vi "subFixUpLooseFiles.vi"(8 "error in (no error)":errorcluster, 9 "Loose files":path[](array[path])=[path "E:/Repos/LVDependencyInspector/obj/DependencyInspector.vi"], 10 "Dependency order":T1[](array[typedef])=[{"Library ref"=refnum, "Target path"=path "E:/Repos/LVDependencyInspector/obj/Addons/LabVIEWObjectInterfaces.lvlibp", "Source name"="LabVIEWObjectInterfaces.lvlib", "Build spec name"="LabVIEWObjectInterfaces"}, {"Library ref"=refnum, "Target path"=path "E:/Repos/LVDependencyInspector/obj/Addons/ErrorManager.lvlibp", "Source name"="ErrorManager.lvlib", "Build spec name"="ErrorManager"}, {"Library ref"=refnum, "Target path"=path "E:/Repos/LVDependencyInspector/obj/Addons/ExtensionInterfaces.lvlibp", "Source name"="ExtensionInterfaces.lvlib", "Build spec name"="ExtensionInterfaces"}, {"Library ref"=refnum, "Target path"=path "E:/Repos/LVDependencyInspector/obj/Addons/LabVIEWItem.lvlibp", "Source name"="LabVIEWItem.lvlib", "Build spec name"="LabVIEWItem"}, {"Library ref"=refnum, "Target path"=path "E:/Repos/LVDependencyInspector/obj/Addons/DefaultExtensions.lvlibp", "Source name"="DefaultExtensions.lvlib", "Build spec name"="DefaultExtensions"}, {"Library ref"=refnum, "Target path"=path "E:/Repos/LVDependencyInspector/obj/Addons/LabVIEWContainers.lvlibp", "Source name"="LabVIEWContainers.lvlib", "Build spec name"="LabVIEWContainers"}, {"Library ref"=refnum, "Target path"=path "E:/Repos/LVDependencyInspector/obj/Addons/LabVIEWFiles.lvlibp", "Source name"="LabVIEWFiles.lvlib", "Build spec name"="LabVIEWFiles"}, {"Library ref"=refnum, "Target path"=path "E:/Repos/LVDependencyInspector/obj/Addons/LabVIEWObjectFactory.lvlibp", "Source name"="LabVIEWObjectFactory.lvlib", "Build spec name"="LabVIEWObjectFactory"}, {"Library ref"=refnum, "Target path"=path "E:/Repos/LVDependencyInspector/obj/Addons/DependencyInspection.lvlibp", "Source name"="DependencyInspection.lvlib", "Build spec name"="DependencyInspection"}, {"Library ref"=refnum, "Target path"=path "E:/Repos/LVDependencyInspector/obj/Addons/DependencyInspector.lvlibp", "Source name"="DependencyInspector.lvlib", "Build spec name"="DependencyInspector"}, {"Library ref"=refnum, "Target path"=path "", "Source name"="Application", "Build spec name"="Application"}], 11 "Local Host App Instance":refnum<vi>) -> (0 "error out":errorcluster)   [LabVIEW 2020, in "SolutionBuilder.lvlib" / "SolutionBuilder.lvclass"]
uses:
  SolutionBuilder.lvclass
  Private/FileInfo.ctl
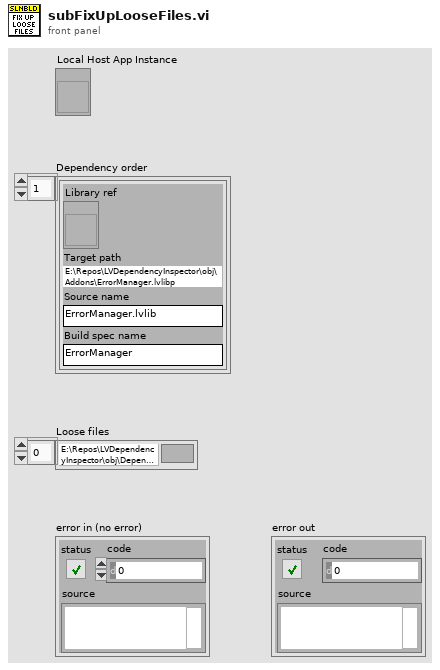
[diagram p1: front panel]
types:
  T1 = typedef "SolutionBuilder.lvlib/SolutionBuilder.lvclass/FileInfo.ctl" = cluster{"Library ref":refnum<vi>, "Target path":path, "Source name":string, "Build spec name":string}
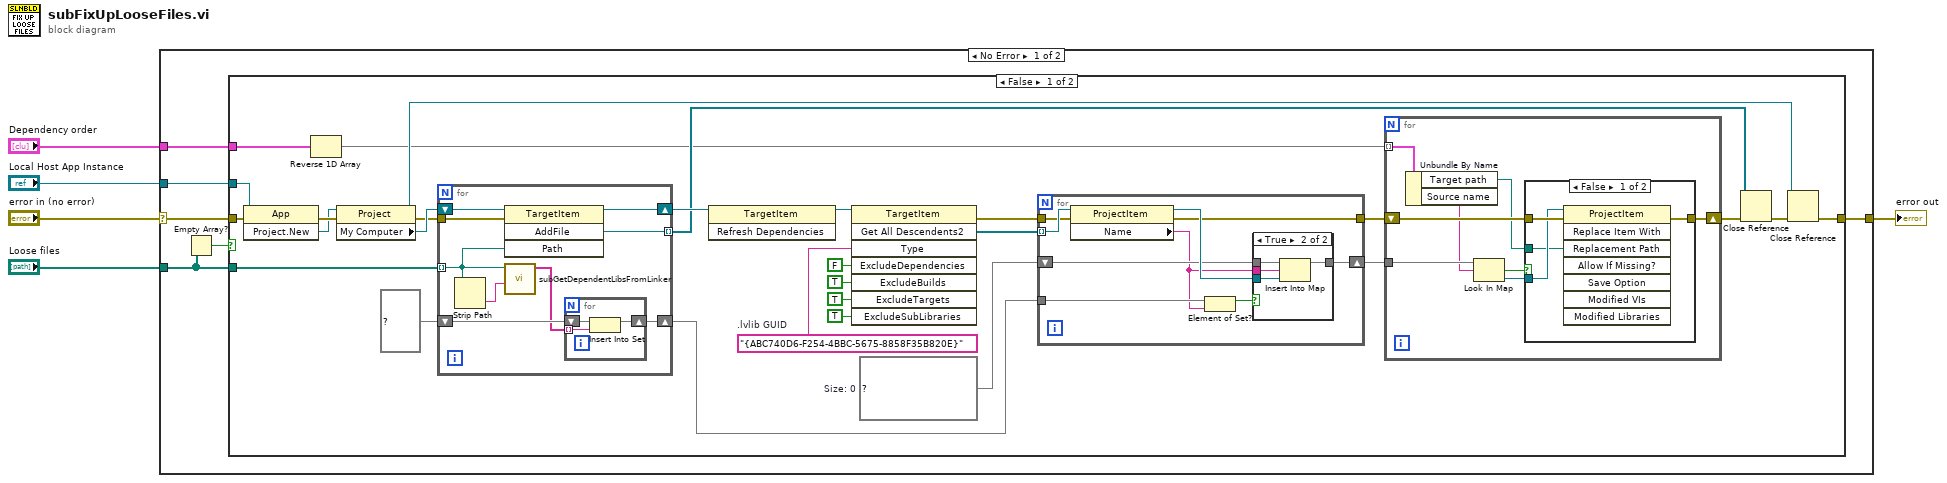
[diagram p0: block diagram]
diagram:
  n1 = case shown="No Error" "error in (no error)" {
    selector: "error in (no error)" -> [w9 w80]
    tunnel: "Loose files" -> [w8 _]
    tunnel: "Dependency order" -> [w11 _]
    tunnel: [w10 w80] -> w3
    tunnel: "Local Host App Instance" -> [w6 _]
    frame No Error {
      n2 = Empty Array?(array=w8) -> (empty?=w7:bool)
      n3 = case shown="False" w7 {
        tunnel: w8 -> [w39 _]
        tunnel: w11 -> [w38 _]
        tunnel: [w37 w79] -> w10
        tunnel: w9 -> [w13 w79]
        tunnel: w6 -> [w12 _]
        frame False {
          w17 = map{string, refnum<vi>} {}  # Size: 0
          w25 = "{ABC740D6-F254-4BBC-5675-8858F35B820E}"  # .lvlib GUID
          n4 = invoke class="App" method="Project.New"(reference=w12, error in=w13) -> (error out=w35:errorcluster, "Project:New"=w29:refnum<vi>)  [unwired: 1 in, 1 out]
          n5 = Reverse 1D Array(array=w38) -> (reversed array=w27:T1[])
          n6 = property class="Project"(reference=w29, error in=w35) -> (reference out=w32:refnum<vi>, error out=w34:errorcluster, "My Computer"=w36:refnum<vi>)
          n7 = for {
            tunnel: w34 -> [w47]
            tunnel: w39 -> [w44] mode=indexing
            tunnel: [w46] -> w30 mode=indexing
            shift-right: [w45] -> w31
            shift-left: w36 -> [w48]
            shift-right: [w42] -> w14
            shift-left: set{string} {} ("set in") -> [w41]
            n8 = Strip Path(path=w44) -> (name=w43:string)  [unwired: 1 out]
            n9 = invoke class="TargetItem" method="AddFile"(reference=w48, error in=w47, "Path"=w44) -> (reference out=w45:refnum<vi>, "AddFile"=w46:refnum<vi>)  [unwired: 1 in, 2 out]
            n10 = call "subGetDependentLibsFromLinker.vi"("Name"=w43, "Path"=w44) -> ("Dependent libs"=w40:string[])  [unwired: 9 in]
            n11 = for {
              shift-right: [w51] -> w42
              shift-left: w41 -> [w50]
              tunnel: w40 -> [w49] mode=indexing
              n12 = Insert Into Set(10:w49, 11:w50) -> (3:w51:set{string})  [unwired: 1 out]
            }
          }
          n13 = invoke class="TargetItem" method="Refresh Dependencies"(reference=w31) -> (reference out=w20:refnum<vi>)  [unwired: 2 in, 2 out]
          n14 = invoke class="TargetItem" method="Get All Descendents2"(reference=w20, "Type"=w25, "ExcludeDependencies"=FALSE, "ExcludeBuilds"=TRUE, "ExcludeTargets"=TRUE, "ExcludeSubLibraries"=TRUE) -> (error out=w19:errorcluster, "Get All Descendents2"=w18:refnum<vi>[])  [unwired: 2 in, 6 out]
          n15 = for {
            tunnel: w18 -> [w60] mode=indexing
            tunnel: w19 -> [w59]
            shift-right: [w57] -> w16
            shift-left: w17 -> [w56]
            tunnel: [w55] -> w15
            tunnel: w14 -> [w54]
            n16 = property class="ProjectItem"(reference=w60, error in=w59) -> (reference out=w58:refnum<vi>, error out=w55:errorcluster, "Name"=w53:string)
            n17 = Element of Set?(10:w53, 11:w54) -> (3:w52:bool)
            n18 = case shown="True" w52 {
              tunnel: w58 -> [_ w65]
              tunnel: [w61 w64] -> w57
              tunnel: w56 -> [w61 w63]
              tunnel: w53 -> [_ w62]
              frame False {
              }
              frame True {
                n19 = Insert Into Map(map in=w63, key=w62, value=w65) -> (map out=w64:map{string, refnum<vi>})  [unwired: 2 out]
              }
            }
          }
          n20 = for {
            tunnel: w16 -> [w73]
            tunnel: w27 -> [w70] mode=indexing
            shift-right: [w71] -> w28
            shift-left: w15 -> [w72]
            n21 = Unbundle By Name(w70) -> ("Target path"=w66:path, "Source name"=w69:string)
            n22 = Look In Map(map=w73, key=w69) -> (key not found?=w68:bool, value=w67:refnum<vi>)  [unwired: 1 in]
            n23 = case shown="False" w68 {
              tunnel: w72 -> [w77 w78]
              tunnel: [w76 w78] -> w71
              tunnel: w67 -> [w75 _]
              tunnel: w66 -> [w74 _]
              frame False {
                n24 = invoke class="ProjectItem" method="Replace Item With"(reference=w75, error in=w77, "Replacement Path"=w74) -> (error out=w76:errorcluster)  [unwired: 5 in, 7 out]
              }
              frame True {
              }
            }
          }
          n25 = Close Reference(reference=w30, error in (no error)=w28) -> (error out=w33:errorcluster)
          n26 = Close Reference(reference=w32, error in (no error)=w33) -> (error out=w37:errorcluster)
        }
        frame True {
        }
      }
    }
    frame Error {
    }
  }
  "error out" <- w3
